vi "CRYIcon Read.vi"(6 "error in (no error)":errorcluster) -> (0 "error out":errorcluster)   [LabVIEW 2013]
doc: "This VI is designed to show how to use tree control methods and properties to perform the following high-level tasks:\n\n1. Use custom symbols for your tree control items.\n2. Traverse an already existing tree in a breadth-first fashion.\n\nRefer to the block diagram and subVI block diagram for implementation."
uses:
  <vilib>/picture/picture.llb/imagedata.ctl
  CRYMainGlobal.vi
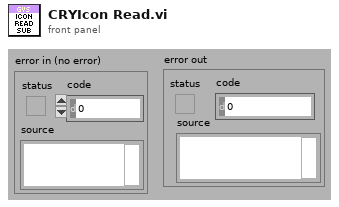
[diagram p1: front panel]
types:
  T1 = typedef "imagedata.ctl" = cluster{"image type":i32, "image depth":i32, "image":u8[], "mask":u8[], "colors":u32[], "Rectangle":cluster{"left":i16, "top":i16, "right":i16, "bottom":i16}}
  T2 = cluster{"left":i16, "top":i16, "right":i16, "bottom":i16}
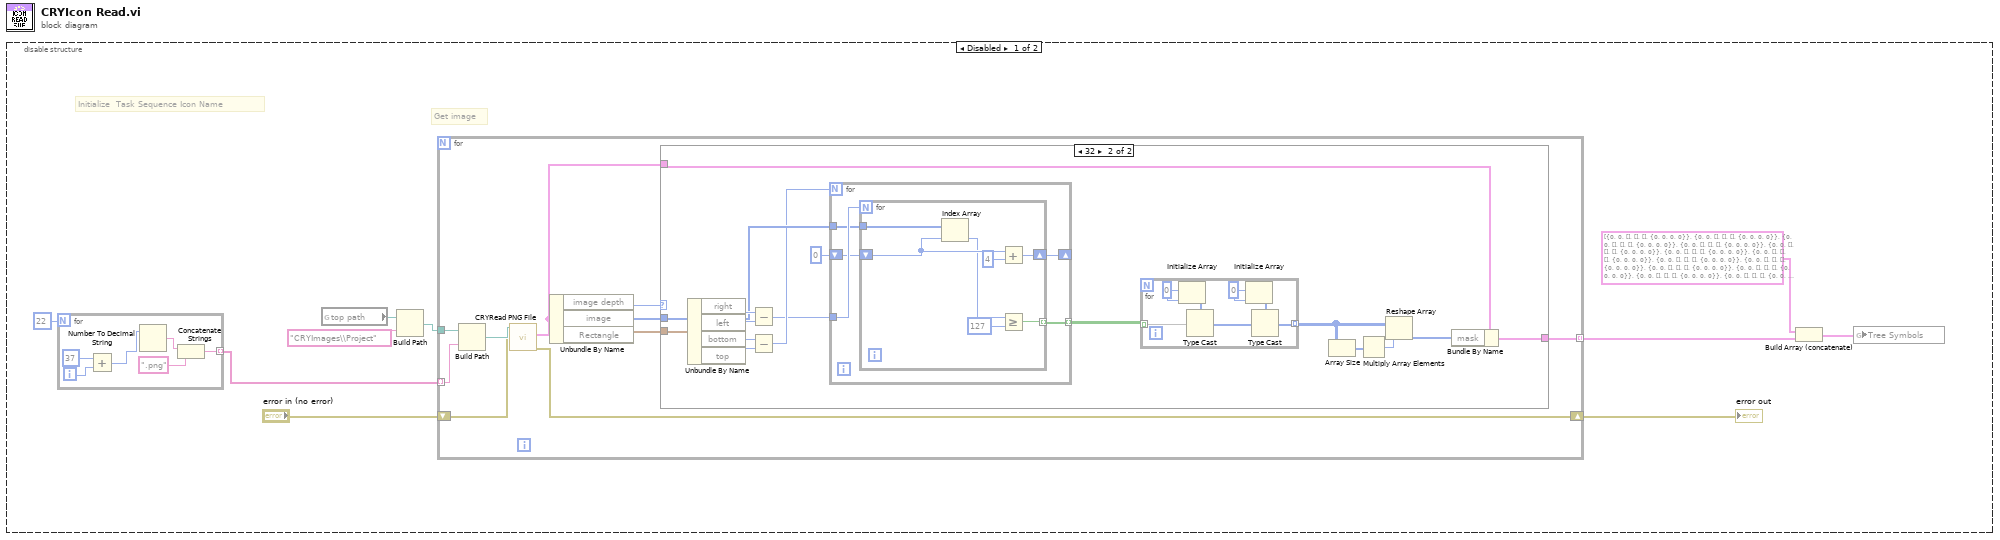
[diagram p0: block diagram]
diagram:
  n1 = disable-structure shown="Disabled" {
    frame Disabled {
      # "Get image"
      # "Initialize  Task Sequence Icon Name"
      n2 = for {
        N: 22 -> [_]
        tunnel: [w13] -> w6 mode=indexing
        i -> [w12]
        n3 = Add(x=37, y=w12) -> (x+y=w11:i32)
        n4 = Number To Decimal String(number=w11) -> (decimal integer string=w15:string)  [unwired: 1 out]
        n5 = Concatenate Strings(w15, ".png" ("string")) -> (w13:string)
      }
      n6 = global read "CRYMainGlobal.vi" "top path"() -> (w1:path)
      n7 = Build Path(base path=w1, name or relative path="CRYImages\\Project") -> (appended path=w2:path)
      n8 = for {
        tunnel: w2 -> [w26]
        tunnel: w6 -> [w25] mode=indexing
        tunnel: [w21] -> w10 mode=indexing
        shift-right: [w17] -> w4
        shift-left: "error in (no error)" -> [w19]
        n9 = Build Path(base path=w26, name or relative path=w25) -> (appended path=w20:path)
        n10 = call "CRYRead PNG File.vi"("error in (no error)"=w19, "path to PNG file"=w20) -> ("error out"=w17:errorcluster, "image data"=w18:T1)  [unwired: 8 out]
        n11 = Unbundle By Name(w18) -> ("image depth"=w22:i32, "image"=w24:u8[], "Rectangle"=w23:T2)
        n12 = case shown="32" w22 {
          tunnel: w23 -> [_ w43]
          tunnel: w24 -> [_ w38]
          tunnel: w18 -> [w27 w29]
          tunnel: [w27 w28] -> w21
          frame Default {
          }
          frame 32 {
            n13 = Unbundle By Name(w43) -> ("right"=w42:i16, "left"=w41:i16, "bottom"=w40:i16, "top"=w39:i16)
            n14 = Subtract(x=w42, y=w41) -> (x-y=w35:i16)
            n15 = Subtract(x=w40, y=w39) -> (x-y=w36:i16)
            n16 = for {
              N: w36 -> [_]
              tunnel: w35 -> [w55]
              tunnel: w38 -> [w54]
              shift-right: [w52] -> _
              shift-left: 0 -> [w53]
              tunnel: [w51] -> w31 mode=indexing
              n17 = for {
                N: w55 -> [_]
                tunnel: w54 -> [w62]
                shift-right: [w61] -> w52
                shift-left: w53 -> [w60]
                tunnel: [w57] -> w51 mode=indexing
                n18 = Index Array(array=w62, index=w60) -> (element=w58:u8)
                n19 = Add(x=w60, y=4) -> (x+y=w61:i32)
                n20 = Greater Or Equal?(x=w58, y=u8 127) -> (x >= y?=w57:bool)
              }
            }
            n21 = for {
              tunnel: [w47] -> w34 mode=indexing
              tunnel: w31 -> [w44] mode=indexing
              w46 = u8 0
              w49 = i16 0
              n22 = Initialize Array(w49, w49) -> (w50:i16[])
              n23 = Type Cast(type=w50, x=w44) -> (*(type *) &x=w48:i16[])
              n24 = Initialize Array(w46, w46) -> (w45:u8[])
              n25 = Type Cast(type=w45, x=w48) -> (*(type *) &x=w47:u8[])
            }
            n26 = Array Size(array=w34) -> (size(s)=w32:i32[])
            n27 = Multiply Array Elements(1:w32) -> (0:w33:i32)
            n28 = Reshape Array(w34, w33) -> (w30:u8[])
            n29 = Bundle By Name(cluster=w29, "mask"=w30) -> (w28:T1)
          }
        }
      }
      "error out" <- w4
      n30 = Build Array (concatenate)(T1[] [{"image type"=0, "image depth"=0, "image"=[], "mask"=[], "colors"=[], "Rectangle"={"left"=0, "top"=0, "right"=0, "bottom"=0}}, {"image type"=0, "image depth"=0, "image"=[], "mask"=[], "colors"=[], "Rectangle"={"left"=0, "top"=0, "right"=0, "bottom"=0}}, {"image type"=0, "image depth"=0, "image"=[], "mask"=[], "colors"=[], "Rectangle"={"left"=0, "top"=0, "right"=0, "bottom"=0}}, {"image type"=0, "image depth"=0, "image"=[], "mask"=[], "colors"=[], "Rectangle"={"left"=0, "top"=0, "right"=0, "bottom"=0}}, {"image type"=0, "image depth"=0, "image"=[], "mask"=[], "colors"=[], "Rectangle"={"left"=0, "top"=0, "right"=0, "bottom"=0}}, {"image type"=0, "image depth"=0, "image"=[], "mask"=[], "colors"=[], "Rectangle"={"left"=0, "top"=0, "right"=0, "bottom"=0}}, {"image type"=0, "image depth"=0, "image"=[], "mask"=[], "colors"=[], "Rectangle"={"left"=0, "top"=0, "right"=0, "bottom"=0}}, {"image type"=0, "image depth"=0, "image"=[], "mask"=[], "colors"=[], "Rectangle"={"left"=0, "top"=0, "right"=0, "bottom"=0}}, {"image type"=0, "image depth"=0, "image"=[], "mask"=[], "colors"=[], "Rectangle"={"left"=0, "top"=0, "right"=0, "bottom"=0}}, {"image type"=0, "image depth"=0, "image"=[], "mask"=[], "colors"=[], "Rectangle"={"left"=0, "top"=0, "right"=0, "bottom"=0}}, {"image type"=0, "image depth"=0, "image"=[], "mask"=[], "colors"=[], "Rectangle"={"left"=0, "top"=0, "right"=0, "bottom"=0}}, {"image type"=0, "image depth"=0, "image"=[], "mask"=[], "colors"=[], "Rectangle"={"left"=0, "top"=0, "right"=0, "bottom"=0}}, {"image type"=0, "image depth"=0, "image"=[], "mask"=[], "colors"=[], "Rectangle"={"left"=0, "top"=0, "right"=0, "bottom"=0}}, {"image type"=0, "image depth"=0, "image"=[], "mask"=[], "colors"=[], "Rectangle"={"left"=0, "top"=0, "right"=0, "bottom"=0}}, {"image type"=0, "image depth"=0, "image"=[], "mask"=[], "colors"=[], "Rectangle"={"left"=0, "top"=0, "right"=0, "bottom"=0}}, {"image type"=0, "image depth"=0, "image"=[], "mask"=[], "colors"=[], "Rectangle"={"left"=0, "top"=0, "right"=0, "bottom"=0}}, {"image type"=0, "image depth"=0, "image"=[], "mask"=[], "colors"=[], "Rectangle"={"left"=0, "top"=0, "right"=0, "bottom"=0}}, {"image type"=0, "image depth"=0, "image"=[], "mask"=[], "colors"=[], "Rectangle"={"left"=0, "top"=0, "right"=0, "bottom"=0}}, {"image type"=0, "image depth"=0, "image"=[], "mask"=[], "colors"=[], "Rectangle"={"left"=0, "top"=0, "right"=0, "bottom"=0}}, {"image type"=0, "image depth"=0, "image"=[], "mask"=[], "colors"=[], "Rectangle"={"left"=0, "top"=0, "right"=0, "bottom"=0}}, {"image type"=0, "image depth"=0, "image"=[], "mask"=[], "colors"=[], "Rectangle"={"left"=0, "top"=0, "right"=0, "bottom"=0}}, {"image type"=0, "image depth"=0, "image"=[], "mask"=[], "colors"=[], "Rectangle"={"left"=0, "top"=0, "right"=0, "bottom"=0}}, {"image type"=0, "image depth"=0, "image"=[], "mask"=[], "colors"=[], "Rectangle"={"left"=0, "top"=0, "right"=0, "bottom"=0}}, {"image type"=0, "image depth"=0, "image"=[], "mask"=[], "colors"=[], "Rectangle"={"left"=0, "top"=0, "right"=0, "bottom"=0}}, {"image type"=0, "image depth"=0, "image"=[], "mask"=[], "colors"=[], "Rectangle"={"left"=0, "top"=0, "right"=0, "bottom"=0}}, {"image type"=0, "image depth"=0, "image"=[], "mask"=[], "colors"=[], "Rectangle"={"left"=0, "top"=0, "right"=0, "bottom"=0}}, {"image type"=0, "image depth"=0, "image"=[], "mask"=[], "colors"=[], "Rectangle"={"left"=0, "top"=0, "right"=0, "bottom"=0}}, {"image type"=0, "image depth"=0, "image"=[], "mask"=[], "colors"=[], "Rectangle"={"left"=0, "top"=0, "right"=0, "bottom"=0}}, {"image type"=0, "image depth"=0, "image"=[], "mask"=[], "colors"=[], "Rectangle"={"left"=0, "top"=0, "right"=0, "bottom"=0}}, {"image type"=0, "image depth"=0, "image"=[], "mask"=[], "colors"=[], "Rectangle"={"left"=0, "top"=0, "right"=0, "bottom"=0}}, {"image type"=0, "image depth"=0, "image"=[], "mask"=[], "colors"=[], "Rectangle"={"left"=0, "top"=0, "right"=0, "bottom"=0}}, {"image type"=0, "image depth"=0, "image"=[], "mask"=[], "colors"=[], "Rectangle"={"left"=0, "top"=0, "right"=0, "bottom"=0}}, {"image type"=0, "image depth"=0, "image"=[], "mask"=[], "colors"=[], "Rectangle"={"left"=0, "top"=0, "right"=0, "bottom"=0}}, {"image type"=0, "image depth"=0, "image"=[], "mask"=[], "colors"=[], "Rectangle"={"left"=0, "top"=0, "right"=0, "bottom"=0}}, {"image type"=0, "image depth"=0, "image"=[], "mask"=[], "colors"=[], "Rectangle"={"left"=0, "top"=0, "right"=0, "bottom"=0}}, {"image type"=0, "image depth"=0, "image"=[], "mask"=[], "colors"=[], "Rectangle"={"left"=0, "top"=0, "right"=0, "bottom"=0}}, {"image type"=0, "image depth"=0, "image"=[], "mask"=[], "colors"=[], "Rectangle"={"left"=0, "top"=0, "right"=0, "bottom"=0}}], w10) -> (w5:T1[])
      n31 = global write "CRYMainGlobal.vi" "Tree Symbols"(w5) -> ()
    }
    frame Enabled {
    }
  }
